vi "Constants.vi"() -> ()   [LabVIEW 2016, in "FPGA RM Test Custom Device Shared.lvlib"]
doc: "Use this Global VI to access the GUIDs assigned to the page resources of the Custom Device."
uses:
  FPGA RM Test Custom Device Shared.lvlib
panel:
  in  "Tab Control":enum32{"GUIDS", "Constants", "Properties"}(tab)
  in  "remove test":string="a204db17-eab5-4bb9-80b1-e59c0bd39c90"
  in  "add test":string="fcf888b8-0ce8-443b-9864-6b469d22d368"
  in  "FPGA RM Test Custom Device":string="eb9566fc-7c4d-4f58-94ce-be480dc54b12"
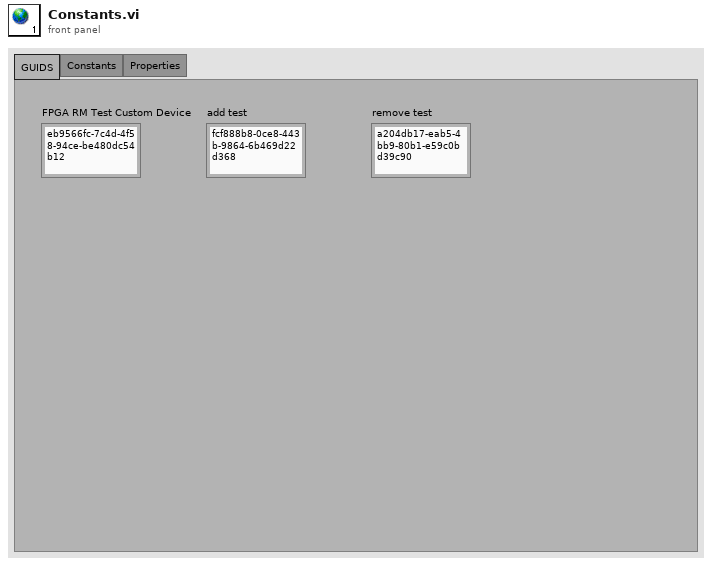
[diagram p1: front panel]
diagram:
